vi "Recompose from Items New.vi"(8 "error in (no error)":errorcluster, 10 "Tree Tag":string, 11 "All Data":refnum<class "Data Item.lvclass">[](array[class])) -> (0 "error out":errorcluster, 2 "XML String":string, 3 "All Data out":refnum<class "Data Item.lvclass">[](array[class]))   [LabVIEW 2026, in "VILab.lvlib"]
uses:
  VILab.lvlib
  Classes/Data Item/Data Item.lvclass
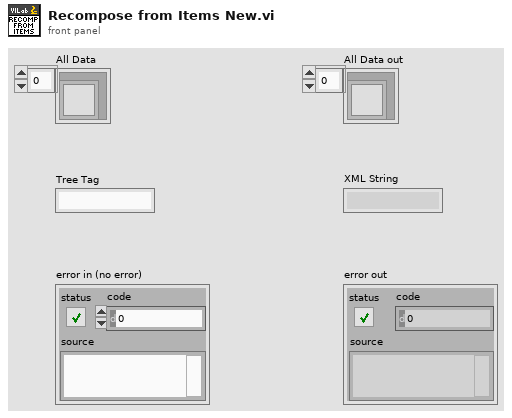
[diagram p1: front panel]
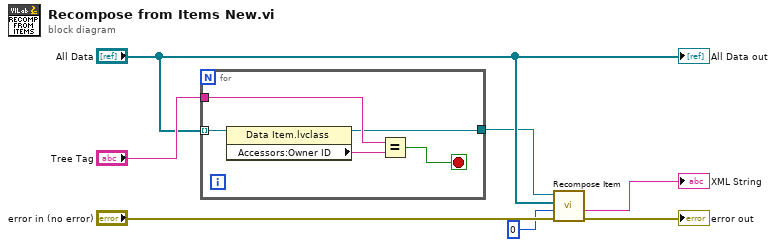
[diagram p0: block diagram]
diagram:
  n1 = for {
    tunnel: "All Data" -> [w12] mode=indexing
    tunnel: "Tree Tag" -> [w10]
    tunnel: [w8] -> w3
    stop <- w9 stop-if-true
    n2 = property class="Data Item.lvclass"(reference=w12) -> (reference out=w8:refnum<class "Data Item.lvclass">, "Accessors:Owner ID"=w11:string)  [unwired: 1 in, 1 out]
    n3 = Equal?(x=w10, y=w11) -> (x = y?=w9:bool)
  }
  n4 = call-dynamic "Recompose Item.vi"("error in (no error)"="error in (no error)", "Nesting Level"=0, "All Data"="All Data", "Data Item in"=w3) -> ("error out"=→"error out":errorcluster, "XML String"=→"XML String":string)  [unwired: 4 in, 2 out]
  "All Data out" <- "All Data"
